vi "Kafka_CreateProducer.vi"(8 "error in (no error)":errorcluster, 9 "Buffer Time (ms)":dbl=100.0, 10 "Topic":string="qamData", 11 "Kafka Broker":string="localhost:9092") -> (0 "error out":errorcluster, 3 "Producer Handle":string)   [LabVIEW 2019, in "LVKafka.lvlib"]
uses:
  LVKafka.lvlib
  KafkaLVLib.dll
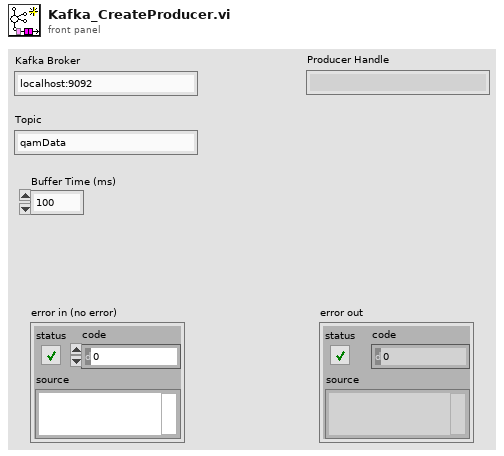
[diagram p1: front panel]
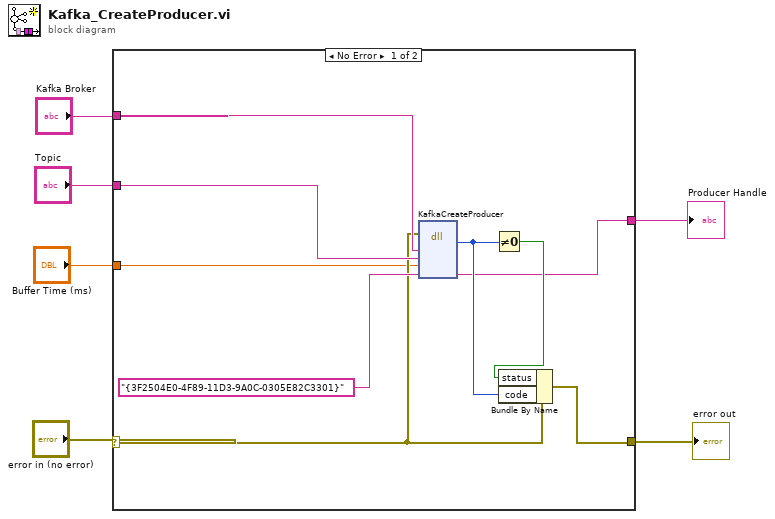
[diagram p0: block diagram]
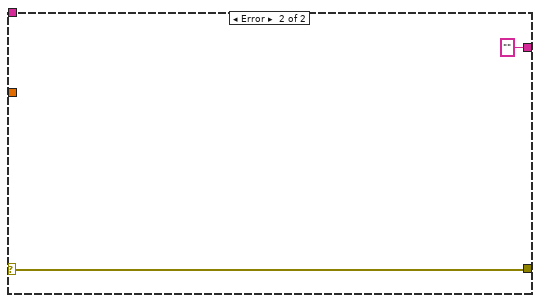
[diagram p2: hidden frame]
diagram:
  n1 = case shown="No Error" "error in (no error)" {
    selector: "error in (no error)" -> [w8 w16]
    tunnel: "Kafka Broker" -> [w12 _]
    tunnel: "Topic" -> [w11 _]
    tunnel: [w13 w16] -> w3
    tunnel: [w9 "" ("consumerHandle")] -> w2
    tunnel: "Buffer Time (ms)" -> [w7 _]
    frame No Error {
      n2 = dll-call lib="KafkaLVLib.*" fn="KafkaCreateProducer"(error in=w8, "kafkaBroker"=w12, "topic"=w11, "bufferingTimeMS"=w7, "producerHandle"="{3F2504E0-4F89-11D3-9A0C-0305E82C3301}" ("consumerHandle")) -> ("error"=w14:i32, "producerHandle"=w9:string)  [unwired: 5 in, 2 out]
      n3 = Not Equal To 0?(x=w14) -> (x != 0?=w15:bool)
      n4 = Bundle By Name(cluster=w8, "status"=w15, "code"=w14) -> (w13:errorcluster)
    }
    frame Error {
    }
  }
  "error out" <- w3
  "Producer Handle" <- w2
